vi "Calculate PID.vi"(1 "scheduling index":i32, 2 "options":T2={"sp low"=0.0, "sp high"=100.0, "out low"=-100.0, "out high"=100.0, "hold (F)"=FALSE, "auto (T)"=TRUE, "pro. band (F)"=FALSE, "reverse acting (T)"=TRUE, "beta"=1.0, "linearity"=1.0, "dt (s)"=-1.0} {"dt (s)" format="%.2f"; "linearity" min=0.0 max=1.0 format="%.2f"; "sp low" format="%.2f"; "sp high" format="%.2f"; "out low" format="%.2f"; "out high" format="%.2f"; "beta" min=0.0 max=1.0 format="%.2f"}, 3 "PID parameters":cluster{"Kc":dbl, "Ti":dbl, "Td":dbl} {"Td" format="%.2f"; "Ti" format="%.2f"; "Kc" format="%.2f"}, 4 "autotuning parameters":T3={"Controller Type"=0, "# of cycles to avg"=3, "Relay amplitude (%)"=0.0, "Control design  "=0, "Noise level %"=0.25} {"Noise level %" format="%.2f"; "Control design" items=["Normal", "Fast", "Slow"]; "Relay amplitude (%)" format="%.2f"; "Controller Type" items=["PID", "PI", "P"]}, 5 "Mean amplitude":dbl format="%.2f", 6 "Mean period":dbl format="%.2f") -> (0 "Tuned PID Parameters":T1 {"Ti" format="%.2f"; "Td" format="%.2f"})   [LabVIEW 2020, in "NI_PID__autopid compat.lvlib"]
doc: "This VI determines the new PID parameters from the results of the setpoint relay experiment."
uses:
  <vilib>/addons/control/pid/NI_PID__autopid compat.lvlib
panel:
  # "Prop Band (%)"
  # "Reset Time (min)"
  # "Deriv Time (min)"
  # "Index"
  # "SP & PV range:"
  # "Output range:"
  # "-1: default,using\nsystem clock"
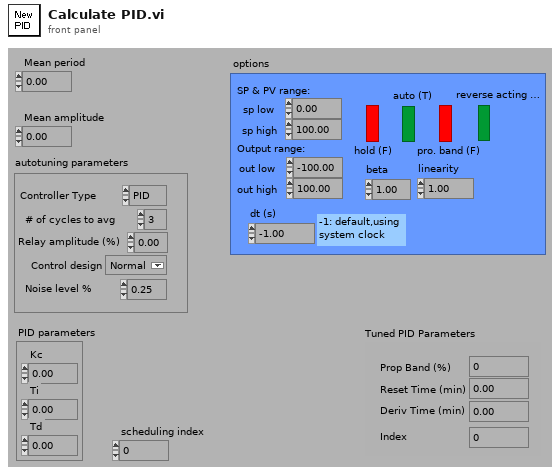
[diagram p1: front panel]
types:
  T1 = cluster{"Kc":dbl, "Ti":dbl, "Td":dbl, "Index":i32}
  T2 = cluster{"sp low":dbl, "sp high":dbl, "out low":dbl, "out high":dbl, "hold (F)":bool, "auto (T)":bool, "pro. band (F)":bool, "reverse acting (T)":bool, "beta":dbl, "linearity":dbl, "dt (s)":dbl}
  T3 = cluster{"Controller Type":u16, "# of cycles to avg":i32, "Relay amplitude (%)":dbl, "Control design  ":u16, "Noise level %":dbl}
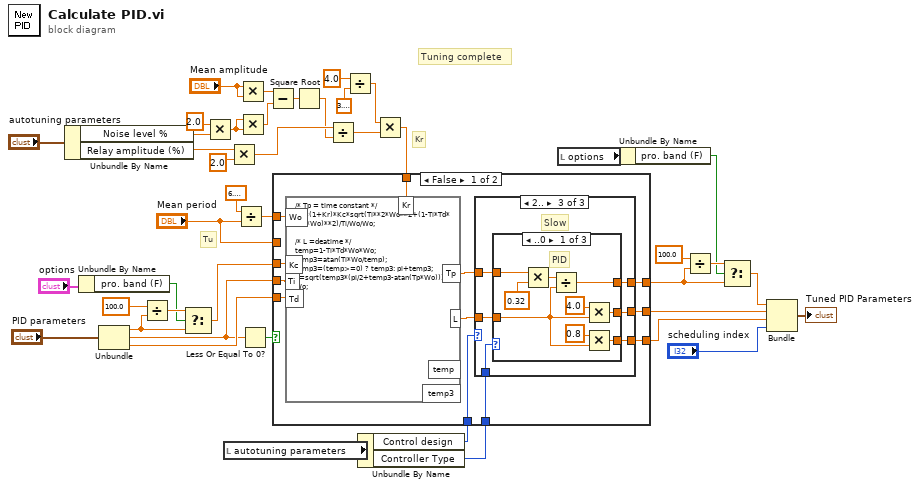
[diagram p0: block diagram]
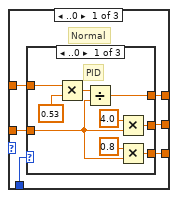
[diagram p2: hidden frame]
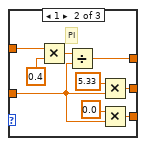
[diagram p3: hidden frame]
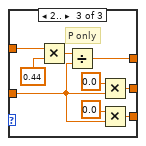
[diagram p4: hidden frame]
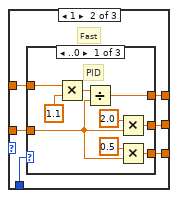
[diagram p5: hidden frame]
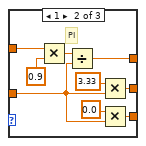
[diagram p6: hidden frame]
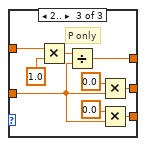
[diagram p7: hidden frame]
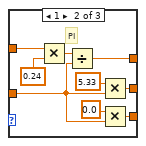
[diagram p8: hidden frame]
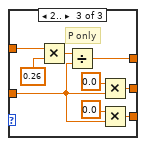
[diagram p9: hidden frame]
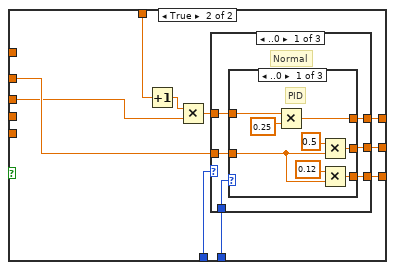
[diagram p10: hidden frame]
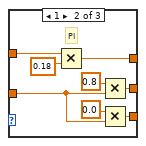
[diagram p11: hidden frame]
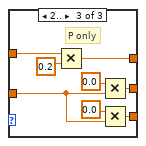
[diagram p12: hidden frame]
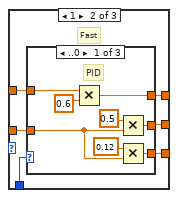
[diagram p13: hidden frame]
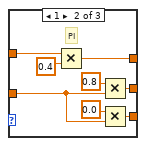
[diagram p14: hidden frame]
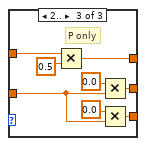
[diagram p15: hidden frame]
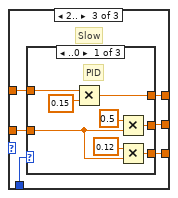
[diagram p16: hidden frame]
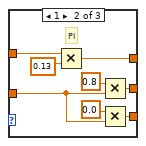
[diagram p17: hidden frame]
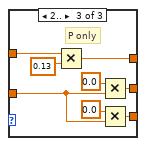
[diagram p18: hidden frame]
diagram:
  # "Tuning complete"
  # "Tu"
  # "Kr"
  n1 = Unbundle By Name("autotuning parameters") -> ("Noise level %"=w12:dbl, "Relay amplitude (%)"=w10:dbl)
  n2 = Unbundle By Name("options") -> ("pro. band (F)"=w17:bool)
  n3 = Unbundle("PID parameters") -> ("Kc"=w23:dbl, "Ti"=w20:dbl, "Td"=w21:dbl)
  n4 = Divide(x=100.0, y=w23) -> (x/y=w24:dbl)
  n5 = Select(t=w24, s=w17, f=w23) -> (s? t:f=w19:dbl)
  n6 = Multiply(x=2.0, y=w12) -> (x*y=w28:dbl)
  n7 = local read "autotuning parameters"() -> (w13:T3)
  n8 = Multiply(x=w10, y=2.0) -> (x*y=w33:dbl)
  n9 = Divide(x=6.283185307179586, y="Mean period") -> (x/y=w3:dbl)
  n10 = Multiply(x="Mean amplitude", y="Mean amplitude") -> (x*y=w30:dbl)
  n11 = Multiply(x=w28, y=w28) -> (x*y=w26:dbl)
  n12 = Less Or Equal To 0?(x=w20) -> (x <= 0?=w40:bool)
  n13 = Subtract(x=w30, y=w26) -> (x-y=w27:dbl)
  n14 = Square Root(x=w27) -> (sqrt(x)=w29:dbl)
  n15 = Divide(x=w33, y=w29) -> (x/y=w31:dbl)
  n16 = Divide(x=4.0, y=3.141592653589793) -> (x/y=w6:dbl)
  n17 = Unbundle By Name(w13) -> ("Control design"=w5:u16, "Controller Type"=w4:u16)
  n18 = Multiply(x=w6, y=w31) -> (x*y=w32:dbl)
  n19 = case shown="False" w40 {
    tunnel: w21 -> [w55 _]
    tunnel: w20 -> [w54 _]
    tunnel: w32 -> [w53 w160]
    tunnel: [w46 w158] -> w38
    tunnel: [w45 w157] -> w25
    tunnel: w19 -> [w52 w155]
    tunnel: w5 -> [w49 w164]
    tunnel: w4 -> [w48 w163]
    tunnel: w3 -> [w47 _]
    tunnel: "Mean period" -> [_ w162]
    tunnel: [w44 w156] -> w1
    frame False {
      n20 = formula code="/* Tp = time constant */\nTp=(1+Kr)*Kc*sqrt(Ti**2*Wo**2+(1-Ti*Td*Wo*Wo)**2)/Ti/Wo/Wo;\n\n/* L =deatime */\ntemp=1-Ti*Td*Wo*Wo;\ntemp3=atan(Ti*Wo/temp);\ntemp3=(temp>=0) ? temp3: pi+temp3;\nL=sqrt(temp3*(pi/2+temp3-atan(Tp*Wo)))/Wo;"("Wo"=w47, "Kr"=w53, "Ti"=w54, "Td"=w55, "Kc"=w52) -> ("Tp"=w50:dbl, "L"=w51:dbl)  [unwired: 2 out]
      n21 = case shown="2.." w49 {
        tunnel: [w61 w90 w125] -> w45
        tunnel: [w60 w91 w126] -> w44
        tunnel: [w59 w92 w127] -> w46
        tunnel: w51 -> [w58 w93 w124]
        tunnel: w50 -> [w57 w94 w123]
        tunnel: w48 -> [w56 w89 w122]
        frame ..0 {
          # "Normal"
          n22 = case shown="..0" w56 {
            tunnel: [w62 w71 w80] -> w59
            tunnel: [w67 w76 w85] -> w61
            tunnel: w58 -> [w66 w75 w84]
            tunnel: [w63 w72 w81] -> w60
            tunnel: w57 -> [w64 w73 w82]
            frame ..0 {
              # "PID"
              n23 = Multiply(x=w64, y=0.53) -> (x*y=w70:dbl)
              n24 = Divide(x=w70, y=w66) -> (x/y=w62:dbl)
              n25 = Multiply(x=4.0, y=w66) -> (x*y=w63:dbl)
              n26 = Multiply(x=0.8, y=w66) -> (x*y=w67:dbl)
            }
            frame 1 {
              # "PI"
              n27 = Multiply(x=w73, y=0.4) -> (x*y=w79:dbl)
              n28 = Divide(x=w79, y=w75) -> (x/y=w71:dbl)
              n29 = Multiply(x=5.33, y=w75) -> (x*y=w72:dbl)
              n30 = Multiply(x=0.0, y=w75) -> (x*y=w76:dbl)
            }
            frame 2.. {
              # "P only"
              n31 = Multiply(x=w82, y=0.44) -> (x*y=w88:dbl)
              n32 = Divide(x=w88, y=w84) -> (x/y=w80:dbl)
              n33 = Multiply(x=0.0, y=w84) -> (x*y=w81:dbl)
              n34 = Multiply(x=0.0, y=w84) -> (x*y=w85:dbl)
            }
          }
        }
        frame 1 {
          # "Fast"
          n35 = case shown="..0" w89 {
            tunnel: [w95 w104 w113] -> w92
            tunnel: [w100 w109 w118] -> w90
            tunnel: w93 -> [w99 w108 w117]
            tunnel: [w96 w105 w114] -> w91
            tunnel: w94 -> [w97 w106 w115]
            frame ..0 {
              # "PID"
              n36 = Multiply(x=w97, y=1.1) -> (x*y=w103:dbl)
              n37 = Divide(x=w103, y=w99) -> (x/y=w95:dbl)
              n38 = Multiply(x=2.0, y=w99) -> (x*y=w96:dbl)
              n39 = Multiply(x=0.5, y=w99) -> (x*y=w100:dbl)
            }
            frame 1 {
              # "PI"
              n40 = Multiply(x=w106, y=0.9) -> (x*y=w112:dbl)
              n41 = Divide(x=w112, y=w108) -> (x/y=w104:dbl)
              n42 = Multiply(x=3.33, y=w108) -> (x*y=w105:dbl)
              n43 = Multiply(x=0.0, y=w108) -> (x*y=w109:dbl)
            }
            frame 2.. {
              # "P only"
              n44 = Multiply(x=w115, y=1.0) -> (x*y=w121:dbl)
              n45 = Divide(x=w121, y=w117) -> (x/y=w113:dbl)
              n46 = Multiply(x=0.0, y=w117) -> (x*y=w114:dbl)
              n47 = Multiply(x=0.0, y=w117) -> (x*y=w118:dbl)
            }
          }
        }
        frame 2.. {
          # "Slow"
          n48 = case shown="..0" w122 {
            tunnel: [w128 w137 w146] -> w127
            tunnel: [w133 w142 w151] -> w125
            tunnel: w124 -> [w132 w141 w150]
            tunnel: [w129 w138 w147] -> w126
            tunnel: w123 -> [w130 w139 w148]
            frame ..0 {
              # "PID"
              n49 = Multiply(x=w130, y=0.32) -> (x*y=w136:dbl)
              n50 = Divide(x=w136, y=w132) -> (x/y=w128:dbl)
              n51 = Multiply(x=4.0, y=w132) -> (x*y=w129:dbl)
              n52 = Multiply(x=0.8, y=w132) -> (x*y=w133:dbl)
            }
            frame 1 {
              # "PI"
              n53 = Multiply(x=w139, y=0.24) -> (x*y=w145:dbl)
              n54 = Divide(x=w145, y=w141) -> (x/y=w137:dbl)
              n55 = Multiply(x=5.33, y=w141) -> (x*y=w138:dbl)
              n56 = Multiply(x=0.0, y=w141) -> (x*y=w142:dbl)
            }
            frame 2.. {
              # "P only"
              n57 = Multiply(x=w148, y=0.26) -> (x*y=w154:dbl)
              n58 = Divide(x=w154, y=w150) -> (x/y=w146:dbl)
              n59 = Multiply(x=0.0, y=w150) -> (x*y=w147:dbl)
              n60 = Multiply(x=0.0, y=w150) -> (x*y=w151:dbl)
            }
          }
        }
      }
    }
    frame True {
      n61 = Increment(x=w160) -> (x+1=w159:dbl)
      n62 = Multiply(x=w159, y=w155) -> (x*y=w161:dbl)
      n63 = case shown="..0" w164 {
        tunnel: [w170 w200 w230] -> w157
        tunnel: [w169 w199 w229] -> w156
        tunnel: [w168 w198 w228] -> w158
        tunnel: w162 -> [w167 w197 w227]
        tunnel: w161 -> [w166 w196 w226]
        tunnel: w163 -> [w165 w195 w225]
        frame ..0 {
          # "Normal"
          n64 = case shown="..0" w165 {
            tunnel: [w171 w179 w187] -> w168
            tunnel: [w176 w184 w192] -> w170
            tunnel: w167 -> [w175 w183 w191]
            tunnel: [w172 w180 w188] -> w169
            tunnel: w166 -> [w173 w181 w189]
            frame ..0 {
              # "PID"
              n65 = Multiply(x=w173, y=0.25) -> (x*y=w171:dbl)
              n66 = Multiply(x=0.5, y=w175) -> (x*y=w172:dbl)
              n67 = Multiply(x=0.12, y=w175) -> (x*y=w176:dbl)
            }
            frame 1 {
              # "PI"
              n68 = Multiply(x=w181, y=0.18) -> (x*y=w179:dbl)
              n69 = Multiply(x=0.8, y=w183) -> (x*y=w180:dbl)
              n70 = Multiply(x=0.0, y=w183) -> (x*y=w184:dbl)
            }
            frame 2.. {
              # "P only"
              n71 = Multiply(x=w189, y=0.2) -> (x*y=w187:dbl)
              n72 = Multiply(x=0.0, y=w191) -> (x*y=w188:dbl)
              n73 = Multiply(x=0.0, y=w191) -> (x*y=w192:dbl)
            }
          }
        }
        frame 1 {
          # "Fast"
          n74 = case shown="..0" w195 {
            tunnel: [w201 w209 w217] -> w198
            tunnel: [w206 w214 w222] -> w200
            tunnel: w197 -> [w205 w213 w221]
            tunnel: [w202 w210 w218] -> w199
            tunnel: w196 -> [w203 w211 w219]
            frame ..0 {
              # "PID"
              n75 = Multiply(x=w203, y=0.6) -> (x*y=w201:dbl)
              n76 = Multiply(x=0.5, y=w205) -> (x*y=w202:dbl)
              n77 = Multiply(x=0.12, y=w205) -> (x*y=w206:dbl)
            }
            frame 1 {
              # "PI"
              n78 = Multiply(x=w211, y=0.4) -> (x*y=w209:dbl)
              n79 = Multiply(x=0.8, y=w213) -> (x*y=w210:dbl)
              n80 = Multiply(x=0.0, y=w213) -> (x*y=w214:dbl)
            }
            frame 2.. {
              # "P only"
              n81 = Multiply(x=w219, y=0.5) -> (x*y=w217:dbl)
              n82 = Multiply(x=0.0, y=w221) -> (x*y=w218:dbl)
              n83 = Multiply(x=0.0, y=w221) -> (x*y=w222:dbl)
            }
          }
        }
        frame 2.. {
          # "Slow"
          n84 = case shown="..0" w225 {
            tunnel: [w231 w239 w247] -> w228
            tunnel: [w236 w244 w252] -> w230
            tunnel: w227 -> [w235 w243 w251]
            tunnel: [w232 w240 w248] -> w229
            tunnel: w226 -> [w233 w241 w249]
            frame ..0 {
              # "PID"
              n85 = Multiply(x=w233, y=0.15) -> (x*y=w231:dbl)
              n86 = Multiply(x=0.5, y=w235) -> (x*y=w232:dbl)
              n87 = Multiply(x=0.12, y=w235) -> (x*y=w236:dbl)
            }
            frame 1 {
              # "PI"
              n88 = Multiply(x=w241, y=0.13) -> (x*y=w239:dbl)
              n89 = Multiply(x=0.8, y=w243) -> (x*y=w240:dbl)
              n90 = Multiply(x=0.0, y=w243) -> (x*y=w244:dbl)
            }
            frame 2.. {
              # "P only"
              n91 = Multiply(x=w249, y=0.13) -> (x*y=w247:dbl)
              n92 = Multiply(x=0.0, y=w251) -> (x*y=w248:dbl)
              n93 = Multiply(x=0.0, y=w251) -> (x*y=w252:dbl)
            }
          }
        }
      }
    }
  }
  n94 = local read "options"() -> (w39:T2)
  n95 = Unbundle By Name(w39) -> ("pro. band (F)"=w34:bool)
  n96 = Divide(x=100.0, y=w38) -> (x/y=w36:dbl)
  n97 = Select(t=w36, s=w34, f=w38) -> (s? t:f=w37:dbl)
  n98 = Bundle(w37, w1, w25, "scheduling index"="scheduling index") -> (→"Tuned PID Parameters":cluster{dbl, dbl, dbl, "scheduling index":i32})  [unwired: 1 out]
